vi "Read Measurements.vi"(8 "error in":errorcluster, 11 "DMM Instrument":refnum<class "DMM Instrument.lvclass">) -> (0 "error out":errorcluster, 2 "Measurements":T1[](array[typedef]) {"Lower limit" format="%#_4p"; "Upper limit" format="%#_4p"}, 3 "DMM Instrument out":refnum<class "DMM Instrument.lvclass">)   [LabVIEW 2025, in "DMM.lvlib" / "DMM Instrument.lvclass"]
uses:
  DMM Instrument.lvclass
  C:/Users/Public/Documents/Sandia National Labs/TSS Plugin/Abstract Engine.lvlibp/Abstract Instrument/Abstract Instrument.lvclass
  Users/Public/Documents/Sandia National Labs/TSS Plugin/Abstract Engine.lvlibp/Abstract Instrument/Channel.ctl
  Users/Public/Documents/Sandia National Labs/TSS Plugin/Abstract Engine.lvlibp/Abstract Instrument/Abstract Instrument.lvclass
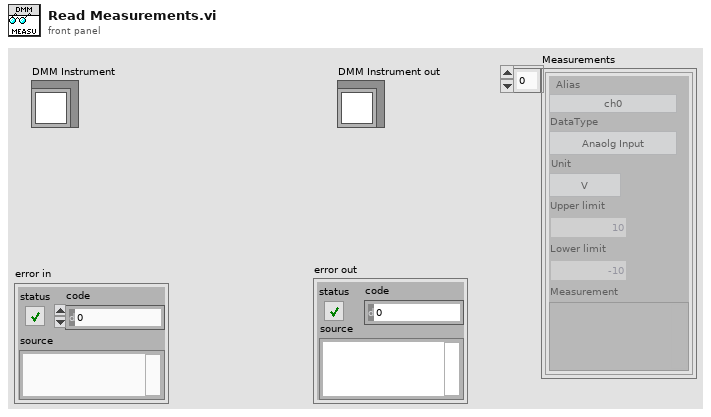
[diagram p1: front panel]
types:
  T1 = typedef "Abstract Engine.lvlibp/Abstract Instrument.lvclass/Channel.ctl" = cluster{"Alias":string, "DataType":enum16{"Anaolg Input", "Waveform"}, "Unit":enum16{"---", "V", "A", "Ohm", "Hz", "uF", "degC", "deg"}, "Upper limit":dbl, "Lower limit":dbl, "Measurement":variant}
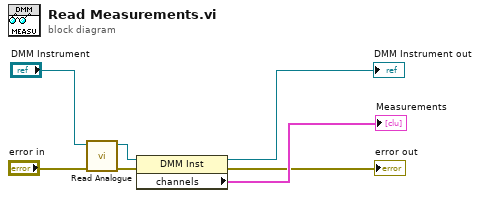
[diagram p0: block diagram]
diagram:
  n1 = call-dynamic "Read Analogue.vi"("error in (no error)"="error in", "Abstract DMM in"="DMM Instrument") -> ("error out"=w5:errorcluster, "Abstract DMM out"=w4:refnum<class "DMM Instrument.lvclass">)  [unwired: 7 in, 1 out]
  n2 = property class="DMM Inst"(reference=w4, error in=w5) -> (reference out=→"DMM Instrument out":refnum<class "DMM Instrument.lvclass">, error out=→"error out":errorcluster, "channels"=→"Measurements":T1[])
